vi "Write Plugin.vi"(7 "id":string, 8 "error in (no error)":errorcluster, 10 "plugin values":T1, 11 "refnum":T3) -> (0 "error out":errorcluster, 2 "replaced?":bool, 3 "refnum out":T3)   [LabVIEW 2017, in "DSF Configuration API.lvlib"]
doc: "Writes a value to a key in a specified section of the configuration data identified by <B>refnum</B>. This VI modifies data in memory. To write data to disk, use the Close Config Data VI. Wire data to the <B>value</B> input to determine the polymorphic instance to use or manually select the instance."
uses:
  DSF Configuration API.lvlib
  Controls/DSF Config Data RefNum.ctl
  Controls/DSF Plugin Info.ctl
  Controls/DSF Timing Info.ctl
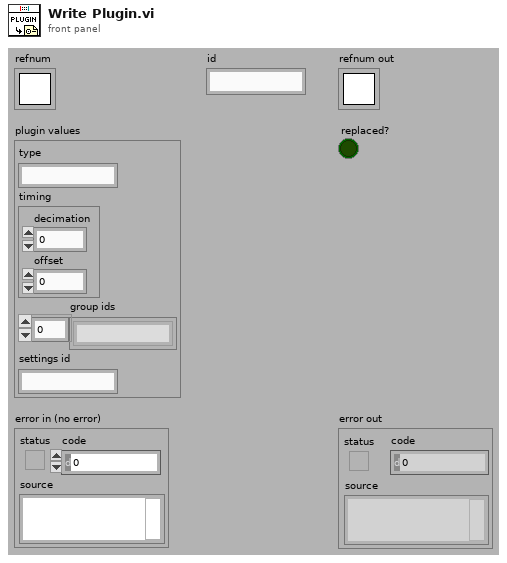
[diagram p1: front panel]
types:
  T1 = typedef "DSF Configuration API.lvlib/DSF Plugin Info.ctl" = cluster{"type":string, "timing":T2, "group ids":string[], "settings id":string}
  T2 = typedef "DSF Configuration API.lvlib/DSF Timing Info.ctl" = cluster{"decimation":i32, "offset":i32}
  T3 = typedef "DSF Configuration API.lvlib/DSF Config Data RefNum.ctl" = refnum<k1>
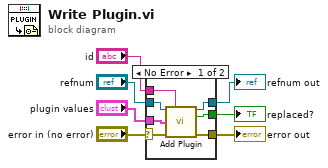
[diagram p0: block diagram]
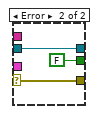
[diagram p2: hidden frame]
diagram:
  n1 = case shown="No Error" "error in (no error)" {
    selector: "error in (no error)" -> [w11 w17]
    tunnel: [w12 w17] -> w6
    tunnel: "id" -> [w14 _]
    tunnel: [w13 FALSE ("key exists?")] -> w4
    tunnel: "refnum" -> [w10 w15]
    tunnel: [w9 w15] -> w2
    tunnel: "plugin values" -> [w8 _]
    frame No Error {
      n2 = call "Add Plugin.vi"("refnum"=w10, "id"=w14, "values"=w8, "error in (no error)"=w11) -> ("refnum out"=w9:T3, "exists?"=w13:bool, "error out"=w12:errorcluster)  [unwired: 2 in, 7 out]
    }
    frame Error {
    }
  }
  "error out" <- w6
  "replaced?" <- w4
  "refnum out" <- w2
